vi "Caterpillar Tester.vi"() -> ()   [LabVIEW 2012]
uses:
  <vilib>/Rock Robotics/WPI/Solenoid/WPI_SolenoidValue.ctl
panel:
  out "Back Leg Cmd":bool
  out "Mid Leg Cmd":enum16{"Down Closed", "Down Opened", "Up"}(ring)
  out "Mid Foot":T1=enum."On"
  in  "Back Leg PS":bool=TRUE
  out "Skids":bool
  out "Front Leg Cmd":enum16{"Down Closed", "Down Opened", "Up"}(ring)
  in  "Back Claws Cmd":bool
  in  "Front Leg Up":bool
  out "Old state 2":string
  out "old state 0":string
  out "Old state 1":string
  in  "Front Claw Cmd":bool
  out "Mid Claw":T1=enum."On"
  out "Back Claw":T1=enum."On"
  out "Front Foot":T1
  out "Front Claw":T1
  out "Current  State":string
  in  "Back Leg Up":bool
  in  "Mid Leg Up":bool
  in  "Mid Leg PS":bool=TRUE
  in  "Front Leg PS":bool=TRUE
  # "Using the Caterpillar Tester\n\nSetup:\n1) Go to Edit menu and click on \n     Reinitialize Values to Default\n2) Click the Run Continuously button\n\nError-Free Climbing:\n1) Click on A (Front Claw Cmd)\n2) Click on B (Back Claws Cmd)\n3) Turn off Front Leg PS button\n4) Turn on Front Leg Up button\n5) Turn on Front Leg PS button\n6) Turn off Front Leg Up button\n7) Turn off Mid Leg PS button\n8) ... needs to be finished ..."
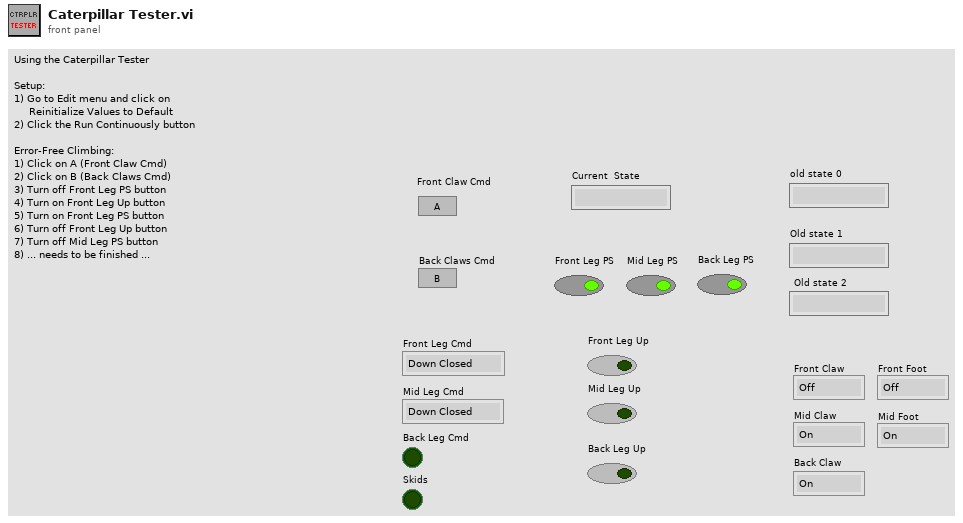
[diagram p1: front panel]
types:
  T1 = typedef "WPI_SolenoidValue.ctl" = enum16{"Off", "On", "Forward", "Reverse"}
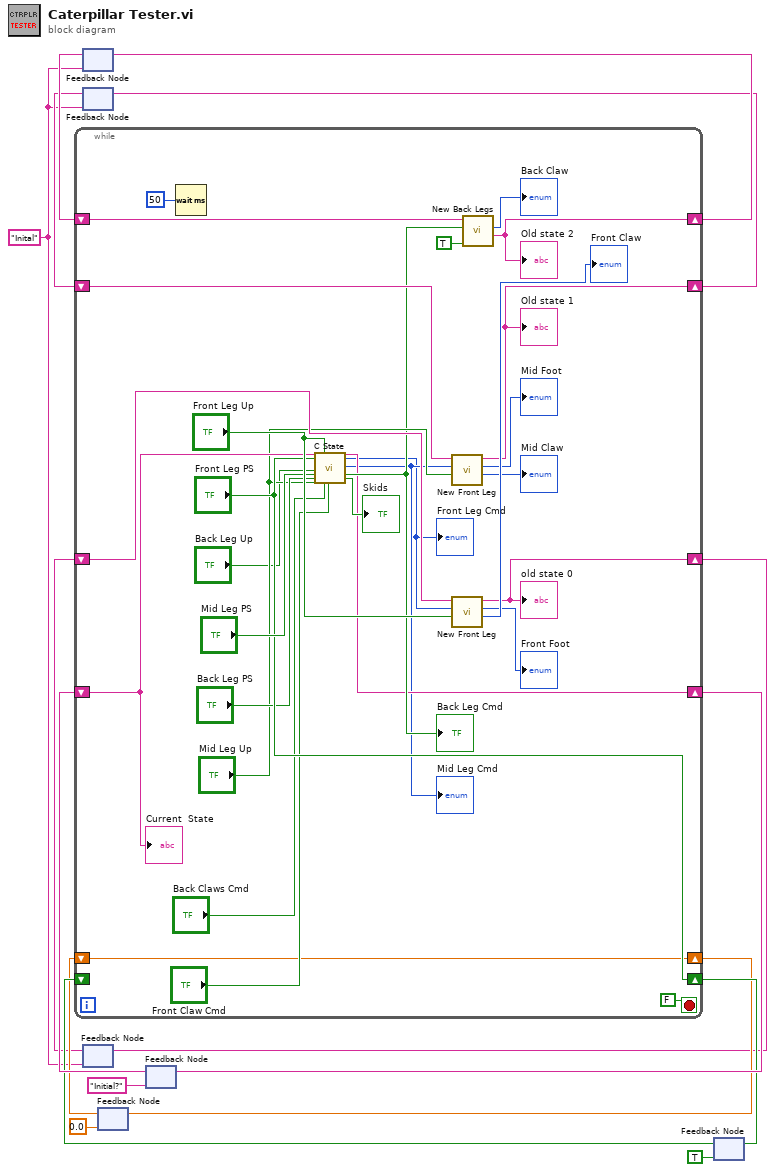
[diagram p0: block diagram]
diagram:
  w1 = "Inital" ("Old state")
  n1 = feedback #1(w1) -> (w6:string)
  n2 = feedback #2(w1) -> (w2:string)
  n3 = feedback #3(w1) -> (w4:string)
  n4 = feedback #4(0.0 ("New Number")) -> (w9:dbl)
  n5 = feedback #5("Initial?" ("New State")) -> (w15:string)
  n6 = feedback #6(TRUE ("New Boolean")) -> (w12:bool)
  n7 = while {
    shift-right: [w20] -> w16
    shift-left: w15 -> [w28]
    shift-right: [w17] -> w10
    shift-left: w9 -> [w17]
    shift-right: ["Front Leg PS"] -> w13
    shift-left: w12 -> [_]
    shift-right: [w37] -> w7
    shift-left: w6 -> [w40]
    shift-right: [w38] -> w5
    shift-left: w4 -> [w39]
    shift-right: [w34] -> w3
    shift-left: w2 -> [w35]
    stop <- FALSE stop-if-true
    n8 = Wait (ms)(milliseconds to wait=u32 50) -> ()  [unwired: 1 out]
    n9 = call "C State.vi"("State"=w28, "Front Leg PS"="Front Leg PS", "Back Leg Up"="Back Leg Up", "Mid Leg PS"="Mid Leg PS", "Back Leg PS"="Back Leg PS", "Mid Leg Up"="Mid Leg Up", "Front Leg Up"="Front Leg Up", "Back Claws Cmd"="Back Claws Cmd", "Front Claw Cmd"="Front Claw Cmd") -> ("newState"=w20:string, "Front Leg Cmd"=w18:enum16{"Down Closed", "Down Opened", "Up"}, "Mid Leg Cmd"=w19:enum16{"Down Closed", "Down Opened", "Up"}, "Engage Back Leg"=w22:bool, "Skids"=→"Skids":bool)  [unwired: 13 in, 1 out]
    "Front Leg Cmd" <- w18
    "Mid Leg Cmd" <- w19
    "Back Leg Cmd" <- w22
    n10 = call "New Front Leg.vi"("Leg up"="Mid Leg Up", "Command"=w19, "Old State"=w35) -> ("Claw"=→"Mid Claw":T1, "Foot"=→"Mid Foot":T1, "New state"=w34:string)  [unwired: 6 in]
    "Old state 1" <- w34
    n11 = call "New Front Leg.vi"("Leg up"="Front Leg Up", "Command"=w18, "Old State"=w39) -> ("Claw"=→"Front Claw":T1, "Foot"=→"Front Foot":T1, "New state"=w38:string)  [unwired: 6 in]
    "old state 0" <- w38
    n12 = call "New Back Legs.vi"("isDualActing"=TRUE, "Engage Leg 1/2"=w22, "New state"=w40) -> ("Old state"=w37:string, "Claw"=→"Back Claw":T1)  [unwired: 7 in]
    "Old state 2" <- w37
    "Current  State" <- w28
  }
  n13 = feedback-in #1(w7) -> ()
  n14 = feedback-in #2(w3) -> ()
  n15 = feedback-in #3(w5) -> ()
  n16 = feedback-in #4(w10) -> ()
  n17 = feedback-in #5(w16) -> ()
  n18 = feedback-in #6(w13) -> ()
